vi "201028_lidar_subVI사용.vi"() -> ()   [LabVIEW 2020]
panel:
  out "Box Point Array":cluster{dbl[], dbl[]}[](array[cluster])
  out "Safe Box Plotting":cluster{dbl[], dbl[]}[](graph)
  out "Clustering graph":T1(graph)
  in  "STOP":bool
  out "XY graph":cluster{"X":dbl, "Y":dbl}[](graph)
  out "XY DATA":cluster{"X":dbl, "Y":dbl}[](array[cluster])
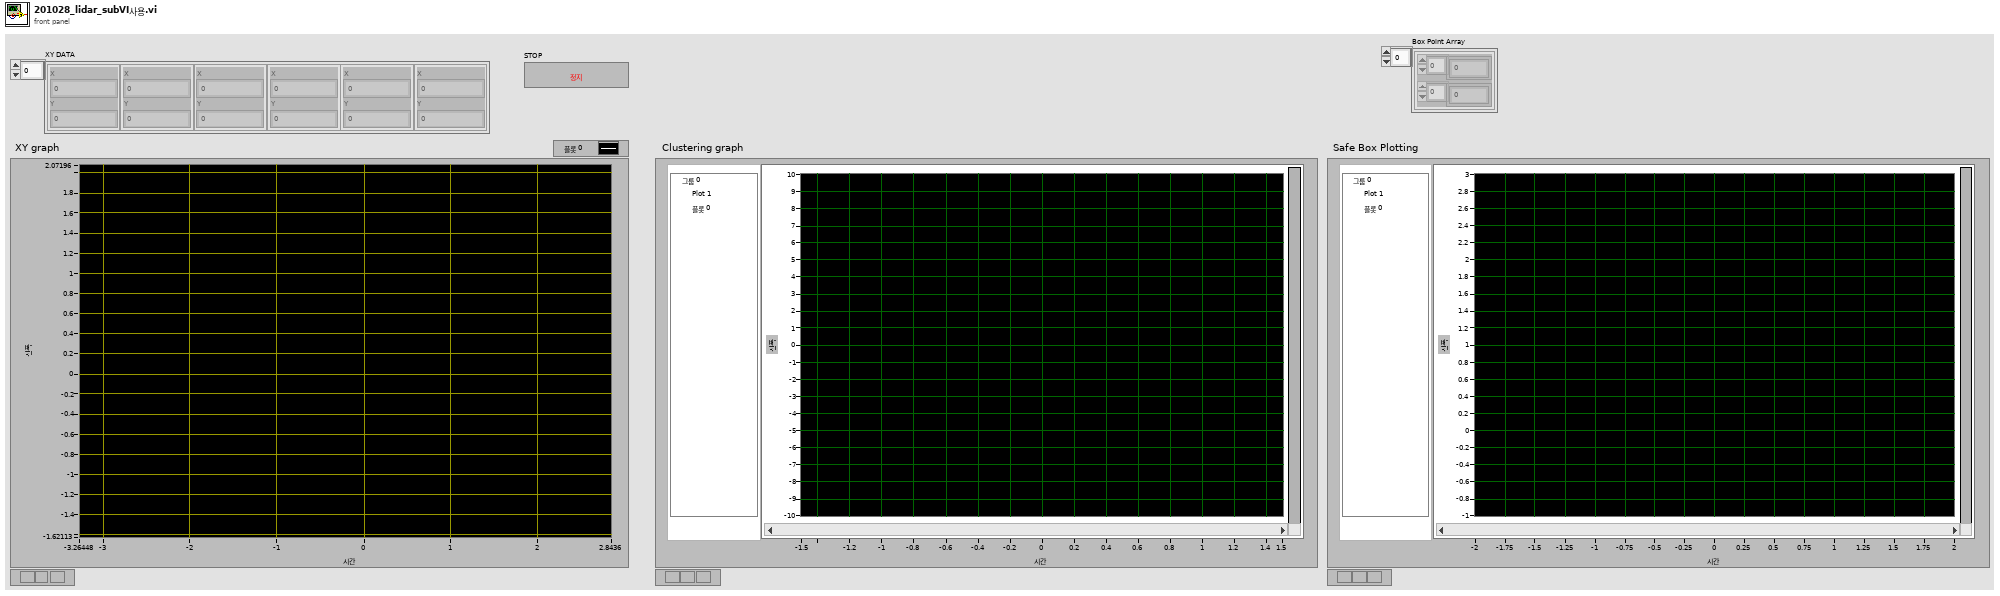
[diagram p1: front panel]
types:
  T1 = cluster{"최종 클러스터링 배열":cluster{"X":dbl, "Y":dbl}[]}[]
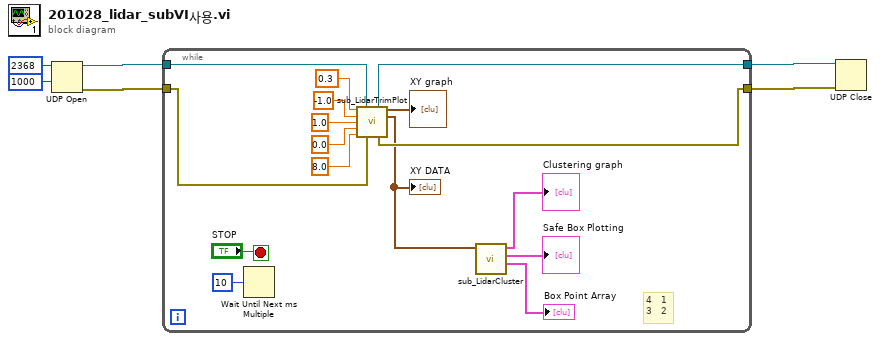
[diagram p0: block diagram]
diagram:
  n1 = UDP Open(9:1000 ("타임아웃 ms (25000)"), 11:u16 2368 ("포트")) -> (port=w3:refnum<k16>, 0:w4:errorcluster)  [unwired: 3 in, 1 out]
  n2 = while {
    tunnel: w3 -> [w15]
    tunnel: w4 -> [w14]
    tunnel: [w13] -> w2
    tunnel: [w12] -> w1
    stop <- "STOP" stop-if-true
    # "4   1\n3   2"
    n3 = Wait Until Next ms Multiple(millisecond multiple=u32 10 ("ms 배수")) -> ()  [unwired: 1 out]
    n4 = call "sub_LidarTrimPlot.vi"("R_min"=0.3, "UDP 네트워크 연결 입력"=w15, "x-"=-1.0, "x+"=1.0, "y-"=0.0, "y+"=8.0, "에러 입력(에러 없음)"=w14) -> ("UDP 네트워크 연결 출력"=w13:refnum<k16>, "Point Cloud Plotting"=→"XY graph":cluster{"X":dbl, "Y":dbl}[], "trim XY DATA"=w10:cluster{"X":dbl, "Y":dbl}[], "에러 출력"=w12:errorcluster)  [unwired: 5 in]
    "XY DATA" <- w10
    n5 = call "sub_LidarCluster.vi"("XY DATA"=w10) -> ("Box Point Array"=→"Box Point Array":cluster{dbl[], dbl[]}[], "Safe Box Plotting"=→"Safe Box Plotting":cluster{dbl[], dbl[]}[], "Cluster Plotting"=→"Clustering graph":T1)  [unwired: 8 in]
  }
  n6 = UDP Close(connection ID=w2, 8:w1) -> ()  [unwired: 2 out]
